vi "Tests the next sequence function.vi"() -> ()   [LabVIEW 2020]
uses:
  Controls/Change setting mode enum.ctl
  Toggle 7/WS1050 1.1/WS1050 1.1.lvclass
  Toggle 6/WS1040/WS1040.lvclass
  Toggle 6/WS1041/WS1041.lvclass
  Toggle 6/WS1042/WS1042.lvclass
  PIC-device/PIC-Device.lvclass
  C:/Sandbox/RF Bench/Source Code/WiSpry Test Framework/Devices/Toggle 6/Toggle 6.lvclass
panel:
  in  "VISA resource name":refnum<visa-resource-name>
  in  "Class to test":enum16{"WS1040", "WS1041", "WS1042"}(ring)
  out "Changes":cluster{"Name":string, "Value":string}[](array[cluster])
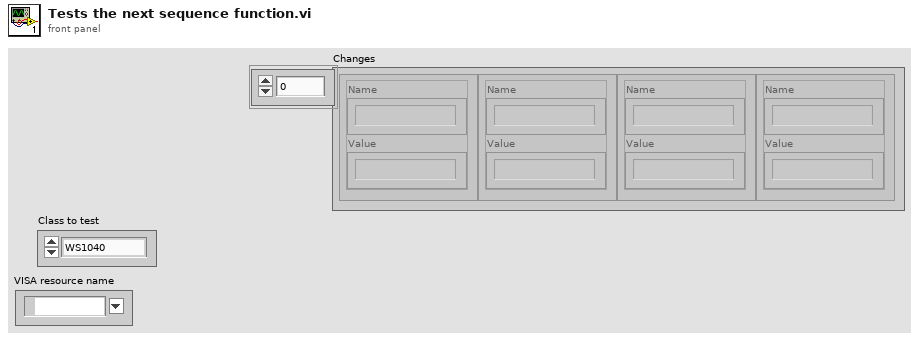
[diagram p1: front panel]
types:
  T1 = typedef "PIC-Device.lvclass/Change setting mode enum.ctl" = enum16{"Init", "Next", "Reset"}
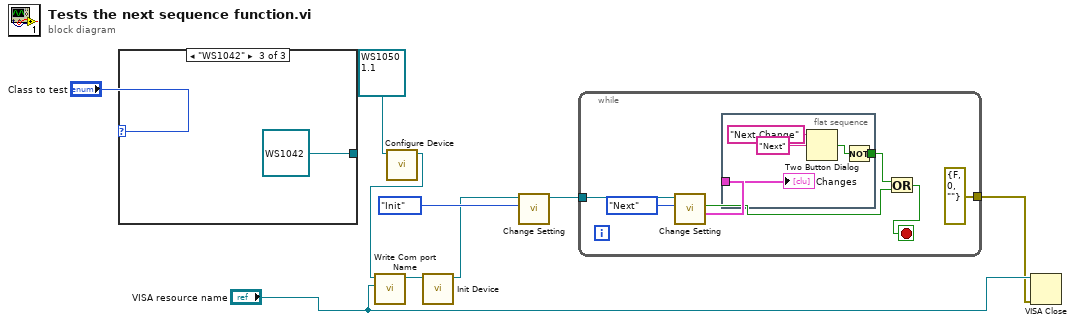
[diagram p0: block diagram]
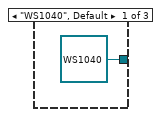
[diagram p2: hidden frame]
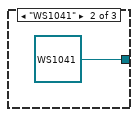
[diagram p3: hidden frame]
diagram:
  n1 = case shown="\"WS1042\"" "Class to test" {
    tunnel: [refnum<class "WS1040.lvclass"> refnum ("WS1040.lvclass") refnum<class "WS1041.lvclass"> refnum ("WS1041.lvclass") refnum<class "WS1042.lvclass"> refnum ("WS1042.lvclass")] -> _
    frame "WS1040", Default {
    }
    frame "WS1041" {
    }
    frame "WS1042" {
    }
  }
  n2 = call-dynamic "Configure Device.vi"("WS1050 1.1 in"=refnum<class "WS1050 1.1.lvclass"> refnum ("WS1050 1.1.lvclass")) -> ("WS1050 1.1 out"=w7:refnum<class "WS1050 1.1.lvclass">)  [unwired: 9 in, 1 out]
  n3 = call-dynamic "Write Com port Name.vi"("Com port Name"="VISA resource name", "Device in"=w7) -> ("Device out"=w6:refnum<class "WS1050 1.1.lvclass">)  [unwired: 9 in]
  n4 = call-dynamic "Init Device.vi"("Toggle 6 in"=w6) -> ("Toggle 6 out"=w1:refnum<class "WS1050 1.1.lvclass">)  [unwired: 9 in, 1 out]
  n5 = call-dynamic "Change Setting.vi"("Change setting mode"=Change_setting_mode_enum."Init", "Toggle 6 in"=w1) -> ("Toggle 6 out"=w9:refnum<class "WS1050 1.1.lvclass">)  [unwired: 6 in, 3 out]
  n6 = while {
    tunnel: w9 -> [w19]
    tunnel: [errorcluster {"status"=FALSE, "code"=0, "source"=""} ("error constant")] -> w2
    stop <- w15 stop-if-true
    n7 = call-dynamic "Change Setting.vi"("Change setting mode"=Change_setting_mode_enum."Next", "Toggle 6 in"=w19) -> ("Changes"=w18:cluster{"Name":string, "Value":string}[], "Last setting"=w16:bool)  [unwired: 6 in, 2 out]
    n8 = flat-sequence {
      tunnel: w18 -> [w24]
      tunnel: [w21] -> w17
      frame #0 {
        n9 = Two Button Dialog(message="Next Change", 2:"Next" ("T button name (\"OK\")")) -> (T button?=w22:bool)  [unwired: 1 in]
        n10 = Not(x=w22) -> (.not. x?=w21:bool)
        "Changes" <- w24
      }
    }
    n11 = Or(x=w17, y=w16) -> (x .or. y?=w15:bool)
  }
  n12 = VISA Close(VISA resource name="VISA resource name", error in (no error)=w2) -> ()  [unwired: 1 out]
